vi "ueye allocate image memory.vi"(0 ".NET (Reference)":refnum<k24>, 5 "Error In":errorcluster) -> (14 "Bits/Pixel 2":i32=8, 15 "Width":i32, 16 "Serial Number":string, 17 "Height":i32, 19 "Error Out":errorcluster)   [LabVIEW 2022 SP3, in "Vision.lvlib"]
uses:
  Vision.lvlib
  C:/Users/Caleb/Desktop/nebraska-silicon-lab/pixel-gantry-control/Gantry/Shared Components/External/bin/uEyeDotNet.dll
  bin/uEyeDotNet.dll
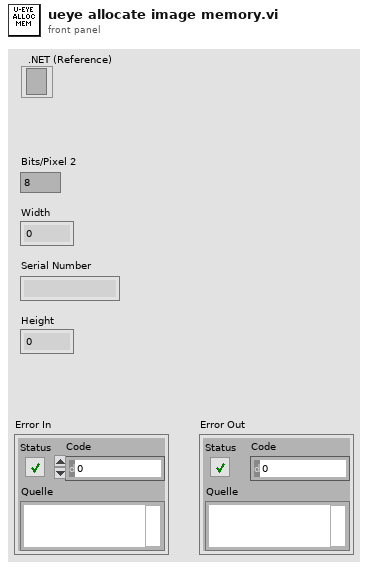
[diagram p1: front panel]
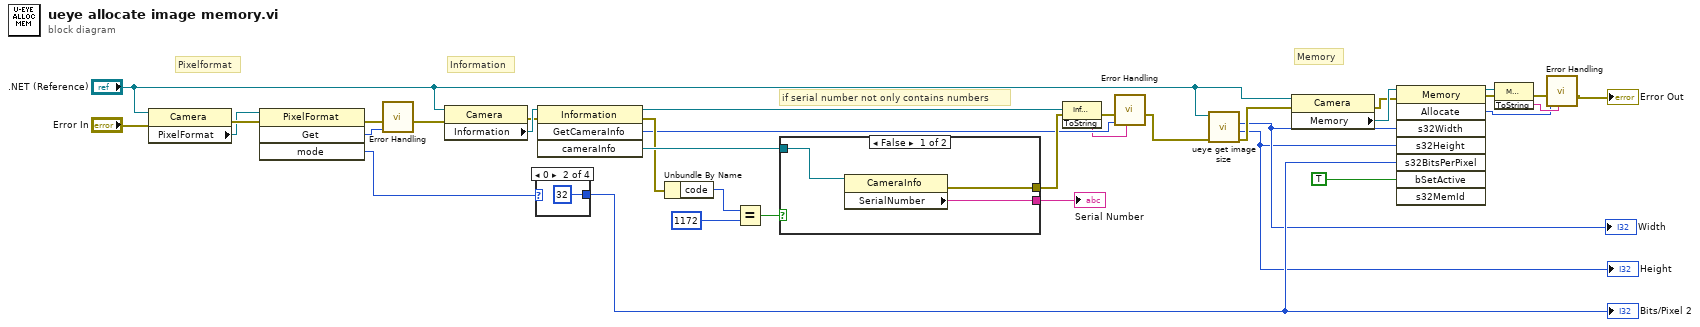
[diagram p0: block diagram]
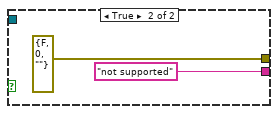
[diagram p2: hidden frame]
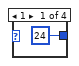
[diagram p3: hidden frame]
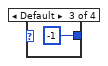
[diagram p4: hidden frame]
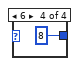
[diagram p5: hidden frame]
diagram:
  # "if serial number not only contains numbers"
  # "Information"
  # "Memory"
  # "Pixelformat"
  n1 = property class="Camera"(reference=".NET (Reference)", error in="Error In") -> (error out=w28:errorcluster, "PixelFormat"=w27:refnum<k24>)  [unwired: 1 out]
  n2 = invoke class="PixelFormat" method="Get"(reference=w27, error in=w28) -> (error out=w14:errorcluster, "Get"=w15:i32, "mode"=w24:i32)  [unwired: 2 in, 1 out]
  n3 = call "Error Handling.vi"("Error Code"=w15, "Error In"=w14) -> ("Error Out"=w13:errorcluster)  [unwired: 9 in]
  n4 = property class="Camera"(reference=".NET (Reference)", error in=w13) -> (error out=w25:errorcluster, "Information"=w26:refnum<k24>)  [unwired: 1 out]
  n5 = case shown="0" w24 {
    tunnel: [24 32 -1 8] -> w32
    frame 1 {
    }
    frame 0 {
    }
    frame Default {
    }
    frame 6 {
    }
  }
  "Bits/Pixel 2" <- w32
  n6 = invoke class="Information" method="GetCameraInfo"(reference=w26, error in=w25) -> (reference out=w35:refnum<k24>, error out=w16:errorcluster, "GetCameraInfo"=w11:i32, "cameraInfo"=w19:refnum<k24>)  [unwired: 2 in]
  n7 = Unbundle By Name(w16) -> ("code"=w20:i32)
  n8 = Equal?(x=w20, y=1172) -> (x = y?=w22:bool)
  n9 = case shown="False" w22 {
    tunnel: [w40 errorcluster {"status"=FALSE, "code"=0, "source"=""} ("Error Out")] -> w17
    tunnel: w19 -> [w42 _]
    tunnel: [w41 "not supported"] -> w18
    frame False {
      n10 = property class="CameraInfo"(reference=w42) -> (error out=w40:errorcluster, "SerialNumber"=w41:string)  [unwired: 1 in, 1 out]
    }
    frame True {
    }
  }
  "Serial Number" <- w18
  n11 = invoke class="Information" method="ToString"(reference=w35, error in=w17) -> (error out=w12:errorcluster, "ToString"=w10:string)  [unwired: 1 in, 1 out]
  n12 = call "Error Handling.vi"("Error String"=w10, "Error Code"=w11, "Error In"=w12) -> ("Error Out"=w9:errorcluster)  [unwired: 8 in]
  n13 = call "ueye get image size.vi"("Error In"=w9, ".NET (Reference)"=".NET (Reference)") -> ("Error Out"=w8:errorcluster, "Height"=w5:i32, "Width"=w6:i32)  [unwired: 6 in, 1 out]
  "Height" <- w5
  "Width" <- w6
  n14 = property class="Camera"(reference=".NET (Reference)", error in=w8) -> (error out=w29:errorcluster, "Memory"=w30:refnum<k24>)  [unwired: 1 out]
  n15 = invoke class="Memory" method="Allocate"(reference=w30, error in=w29, "s32Width"=w6, "s32Height"=w5, "s32BitsPerPixel"=w32, "bSetActive"=TRUE) -> (reference out=w34:refnum<k24>, error out=w33:errorcluster, "Allocate"=w1:i32)  [unwired: 2 in, 5 out]
  n16 = invoke class="Memory" method="ToString"(reference=w34, error in=w33) -> (error out=w4:errorcluster, "ToString"=w2:string)  [unwired: 1 in, 1 out]
  n17 = call "Error Handling.vi"("Error String"=w2, "Error Code"=w1, "Error In"=w4) -> ("Error Out"=→"Error Out":errorcluster)  [unwired: 8 in]
